vi "Main.vi"(8 "error in (no error)":errorcluster, 11 "LineCCD in":refnum<class "LineCCD.lvclass">) -> (0 "error out":errorcluster, 3 "component":refnum<class "LineCCD.lvclass">)   [LabVIEW 2012, in "LineCCD.lvclass"]
doc: "Main VI of the component. This should contain the GUI of your component and be called when creating an executable."
uses:
  LineCCD.lvclass
  <vilib>/Distrio/Murmex/Murmex/command_enum.ctl
  <instrlib>/ALPHALAS CCD S Series/Public/Typedefs/Operating Mode.ctl
  LineCCD.lvclass/LineCCD.ctl
  <vilib>/Distrio/Murmex/InitialiseMessage/InitialiseMessage.lvclass
  <vilib>/Distrio/Murmex/Murmex/update_cluster.ctl
  <vilib>/Distrio/Murmex/GenericMessage/GenericMessage.lvclass
  <vilib>/Distrio/Murmex/TerminateMessage/TerminateMessage.lvclass
  <vilib>/Distrio/Murmex/ConfigureMessage/ConfigureMessage.lvclass
  <vilib>/Distrio/Murmex/StartMessage/run mode enum.ctl
  <vilib>/Distrio/Murmex/StopMessage/StopMessage.lvclass
  <vilib>/Distrio/Murmex/StartMessage/StartMessage.lvclass
  <vilib>/Distrio/Murmex/ResetMessage/ResetMessage.lvclass
  <vilib>/Distrio/Murmex/Murmex/Set configure at initialise.vi
  <vilib>/Distrio/Murmex/Murmex/Set log reference.vi
  <vilib>/Distrio/Murmex/Murmex/Set VI reference.vi
  <vilib>/Distrio/Murmex/Murmex/Get ID.vi
  <vilib>/Distrio/Murmex/Murmex/Set write log to disk.vi
  <vilib>/Distrio/Murmex/Message/Add or replace parameter.vi
  <vilib>/Distrio/Murmex/Murmex/Murmex.lvclass
  <vilib>/Distrio/Murmex/Message/Message.lvclass
  <instrlib>/ALPHALAS CCD S Series/ALPHALAS CCD S Series.lvlib
panel:
  in  "button:single frame":bool
  in  "Tab Control 2":enum32{"Info"}(tab)
  out "frame rate":dbl[unit]
  out "sensor read out time":dbl[unit]
  out "pixels per scan":u32
  out "pixel height":dbl[unit]
  out "pixel width":dbl[unit]
  out "pixel pitch":dbl[unit]
  out "clock speed":dbl[unit]
  out "trigger out control supported":bool
  out "status":string
  in  "button:reset":bool
  out "terminate?":bool
  in  "Tab Control":enum32{"Main", "Debug"}(tab)
  in  "fit data?":bool
  out "delta":dbl[unit]
  in  "Operating Mode":T1 items=["Int Synch, Continuously Running w SW Capture-Start", "Int Synch, Continuously Running w HW Capture-Start", "Int Synch, Continuously Running w HW Capture-Enable", "Single Shot, Clean&Ready w ext. HW Trigger", "Ext Synch, Continuously Runnung w SW Capture-Start"]
  in  "reset background":bool
  in  "background":bool
  out "max":dbl[unit]
  out "max":u32
  out "min integration time":dbl[unit] caption="min"
  out "max integration time":dbl[unit] caption="max"
  in  "calculate average":bool
  in  "Hardware dark \ncorrection":bool
  in  "Enable trig out\nafter config":bool
  in  "Trig out before integration":dbl[unit] max=0.001849
  in  "Scans per Acquisition":u32 max=4599
  in  "Integration time":dbl[unit] min=9.999999999999999e-06 max=60.0 step=1e-06
  out "Line profile":cluster{cdb[]}[](graph)
  in  "button:select ROIs":bool
  in  "button:free run":bool
  in  "save average":bool
  in  "file name":string
  in  "set intercept":bool
  in  "send delta":bool
  out "pixel shift":dbl
  in  "button:configure":bool
  in  "button:quit":bool
  out "LPB":cluster{cdb[]}[](graph)
  out "LPA":cluster{cdb[]}[](graph)
  out "fitting fine?":bool
  out "signal above threshold?":bool
  in  "Component id":string="LineCCD"
  out "log":string
  in  "button:send command":bool
  in  "generic command":string
  in  "command":T2
  # "Settings"
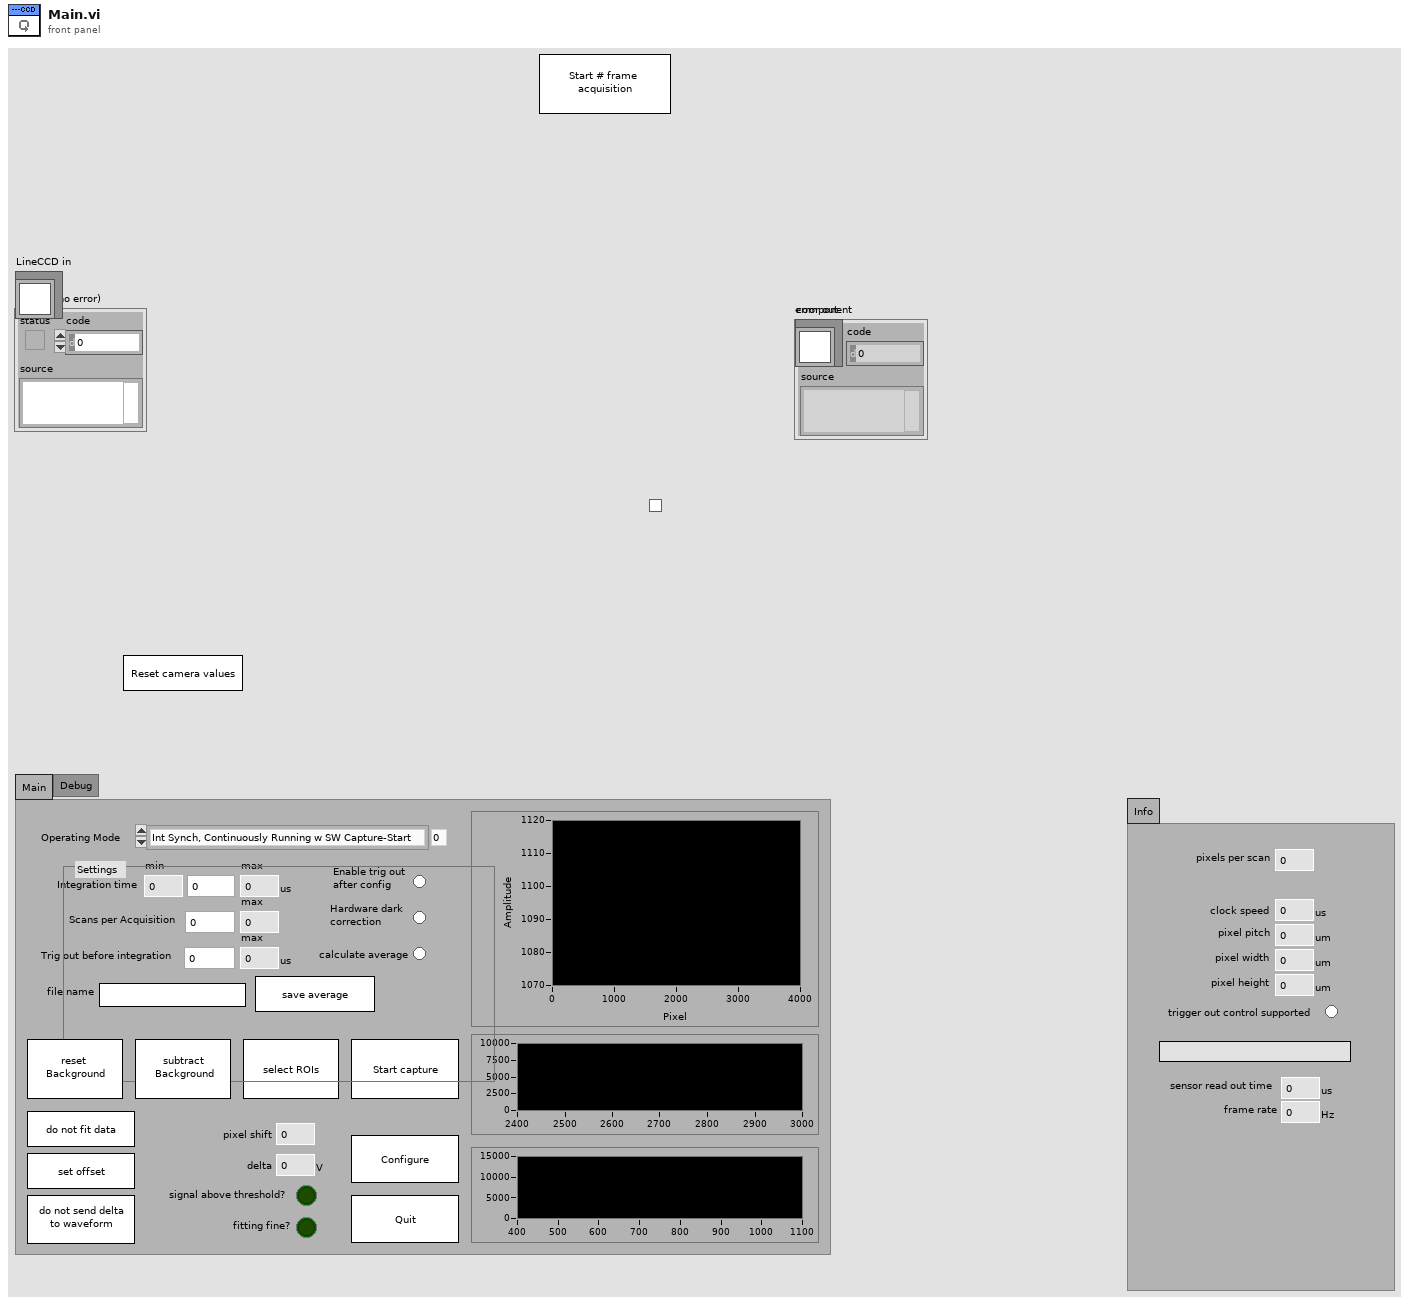
[diagram p1: front panel]
types:
  T1 = typedef "ALPHALAS CCD S Series.lvlib/Operating Mode.ctl" = u16
  T2 = typedef "Murmex.lvlib/Murmex.lvclass/command_enum.ctl" = enum16{"null", "initialise", "reset", "terminate", "acknowledge", "update", "inspect", "inform", "proceed", "start", "stop", "fetch", "configure", "generic"}
  T3 = typedef "Murmex.lvlib/Murmex.lvclass/update_cluster.ctl" = cluster{"target ID":string, "key chains":string[], "values":variant[]}
  T4 = enum8{"Enabled", "Disabled", "Disabled and Grayed Out"}
  T5 = typedef "Murmex.lvlib/StartMessage.lvclass/run mode enum.ctl" = enum16{"infinite", "finite"}
  T6 = typedef "Murmex.lvclass/command_enum.ctl" = enum16{"null", "initialise", "reset", "terminate", "acknowledge", "update", "inspect", "inform", "proceed", "start", "stop", "fetch", "configure", "generic"}
  T7 = typedef "Murmex.lvclass/Event type enumerations.ctl" = enum16{"before", "after"}
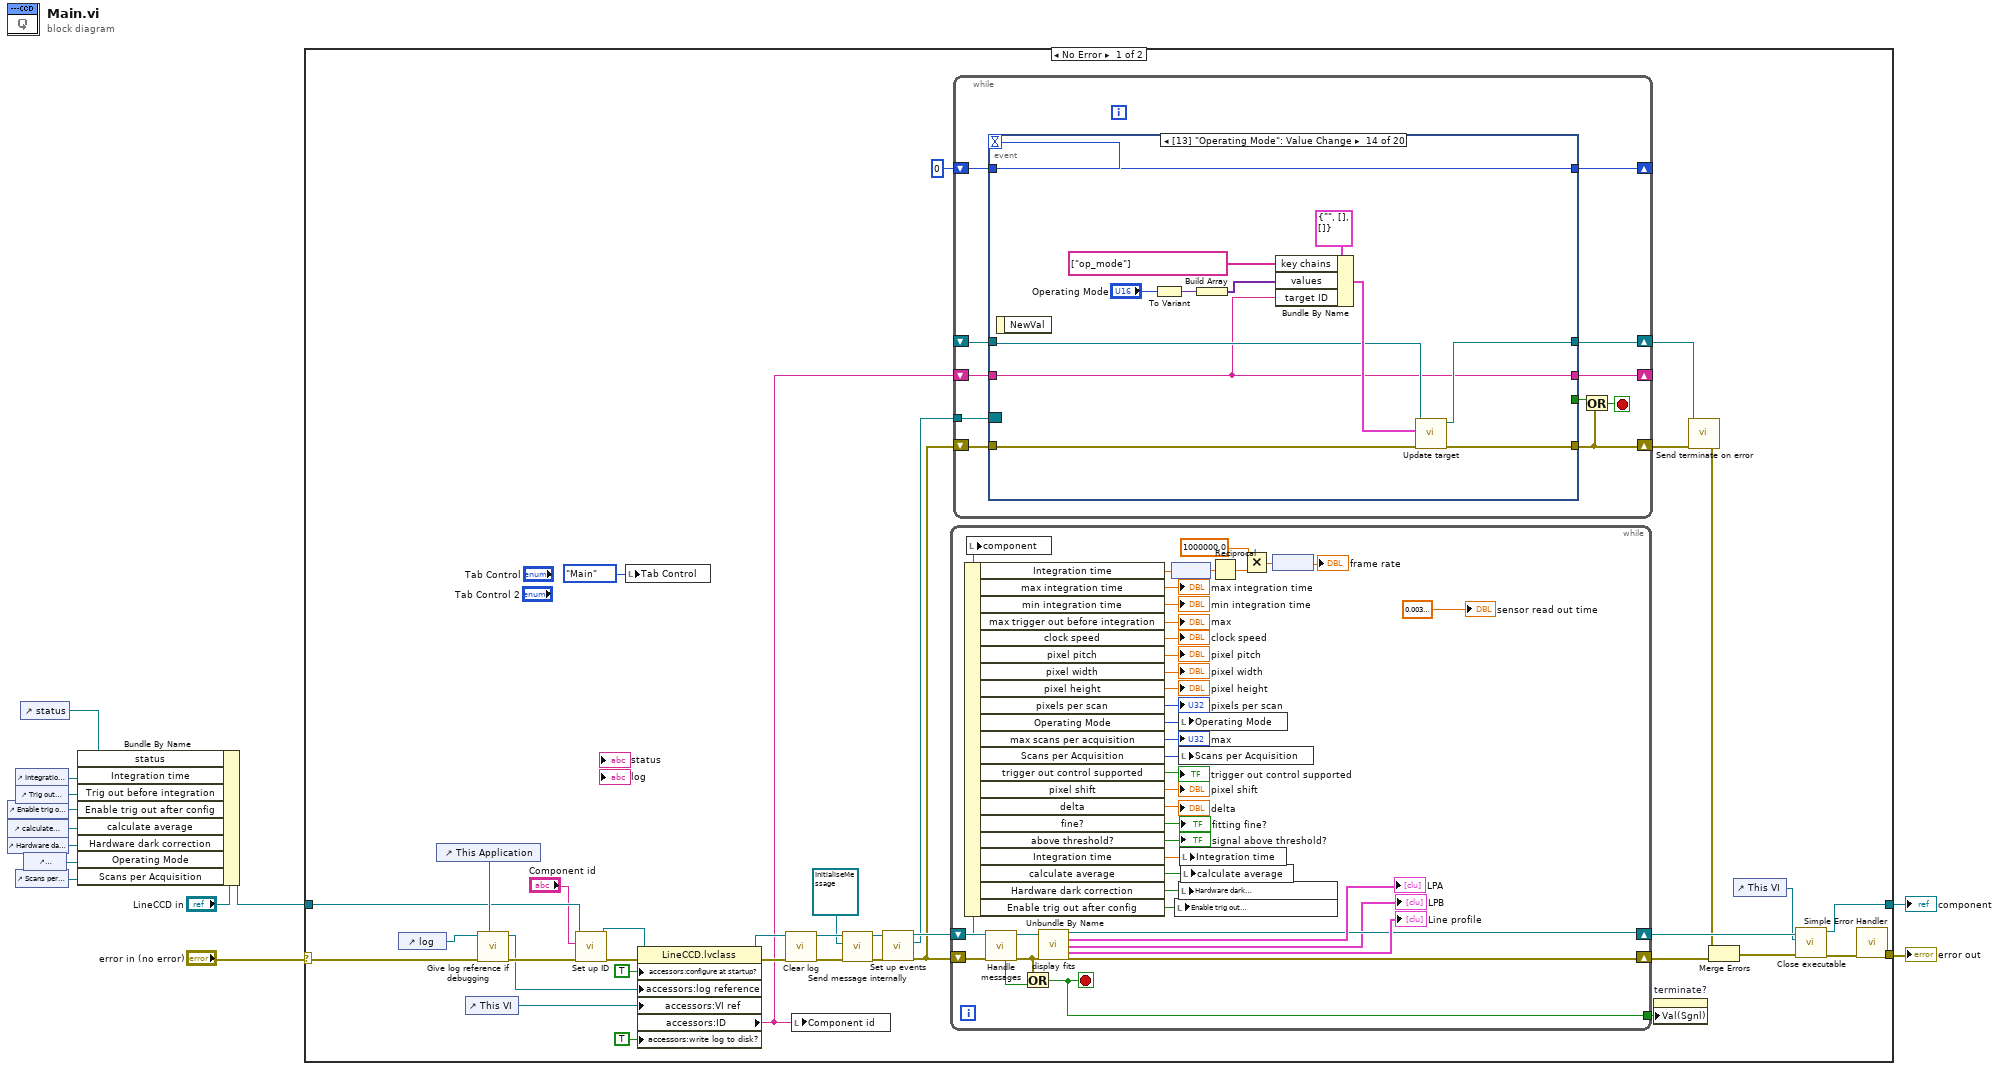
[diagram p0: block diagram]
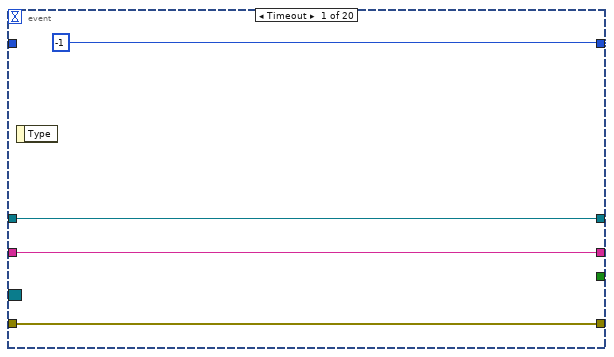
[diagram p2: hidden frame]
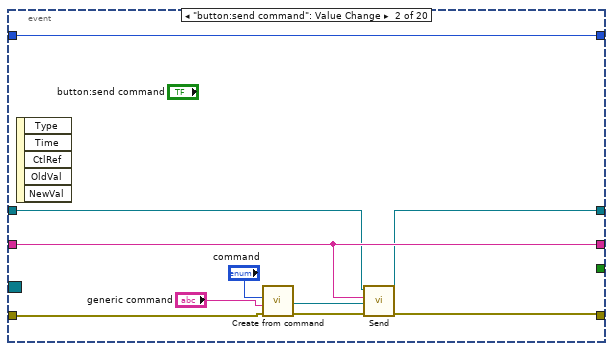
[diagram p3: hidden frame]
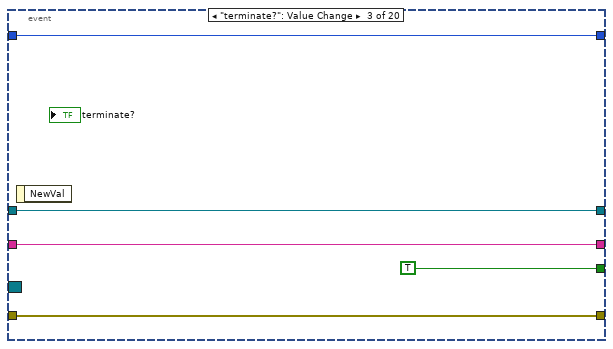
[diagram p4: hidden frame]
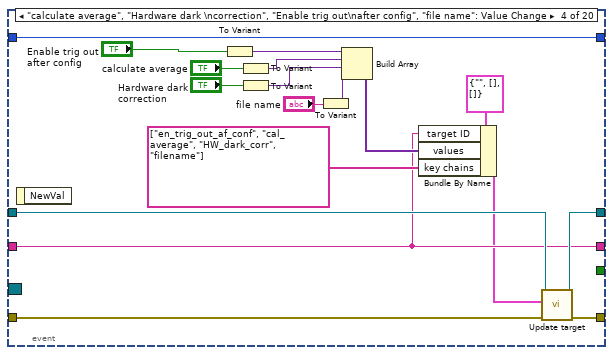
[diagram p5: hidden frame]
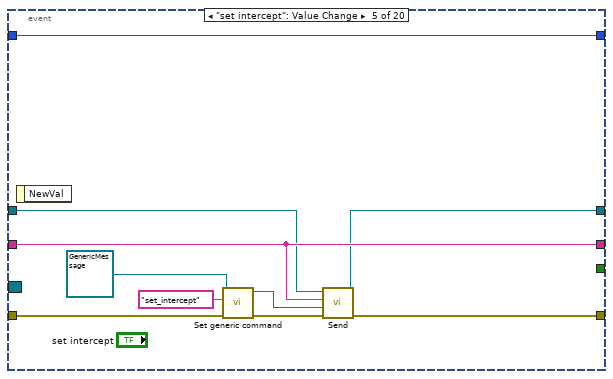
[diagram p6: hidden frame]
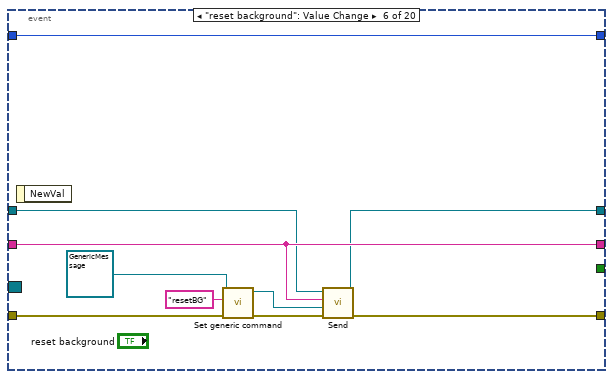
[diagram p7: hidden frame]
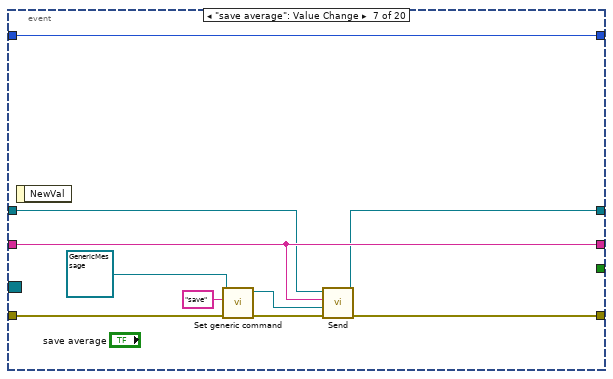
[diagram p8: hidden frame]
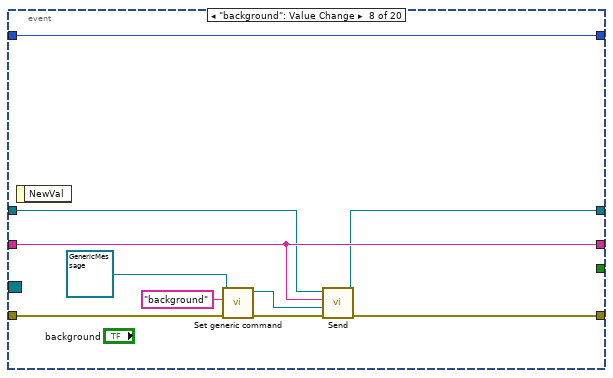
[diagram p9: hidden frame]
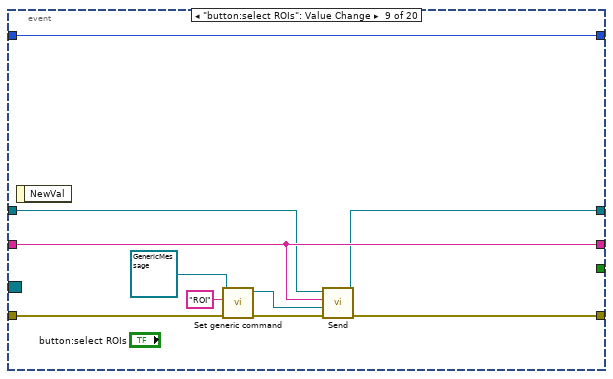
[diagram p10: hidden frame]
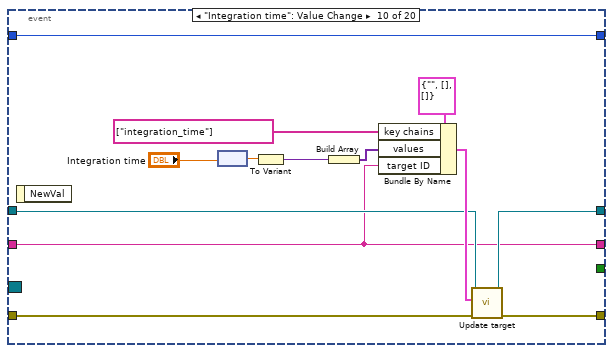
[diagram p11: hidden frame]
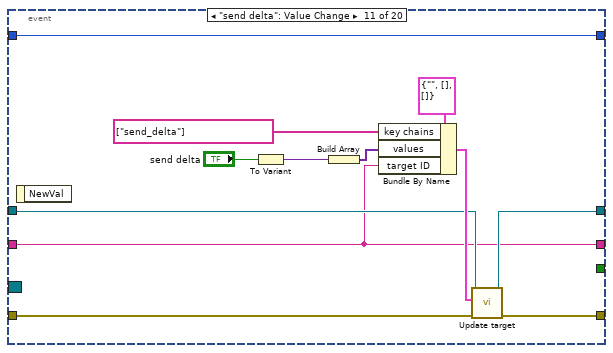
[diagram p12: hidden frame]
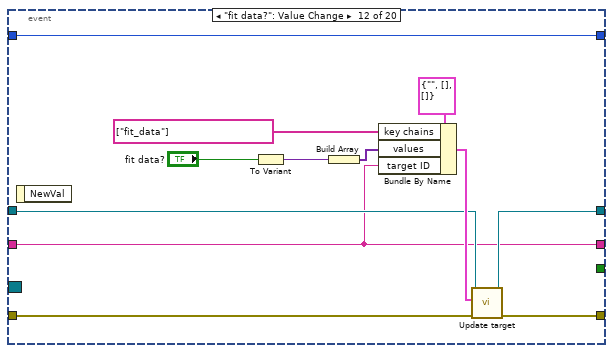
[diagram p13: hidden frame]
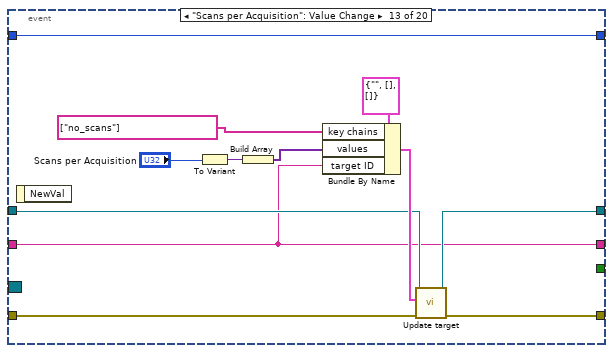
[diagram p14: hidden frame]
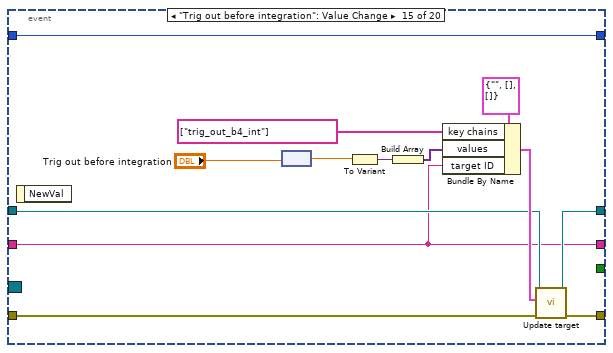
[diagram p15: hidden frame]
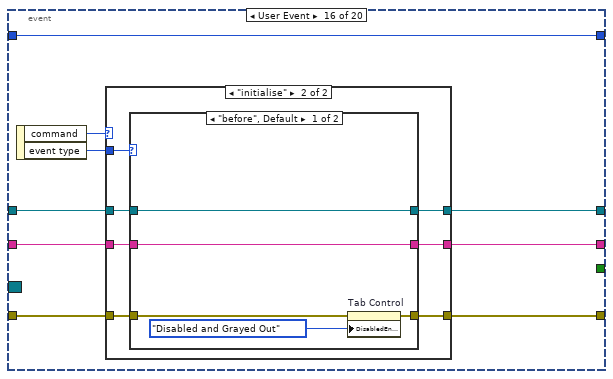
[diagram p16: hidden frame]
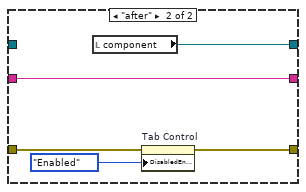
[diagram p18: hidden frame]
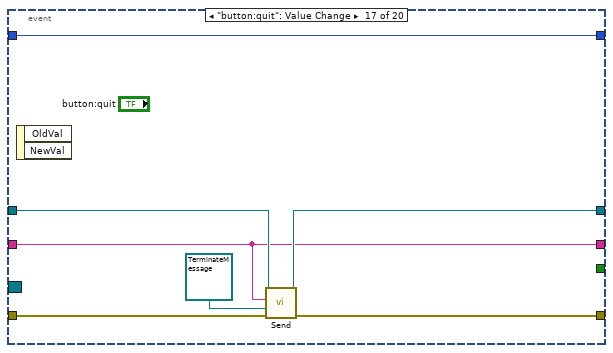
[diagram p19: hidden frame]
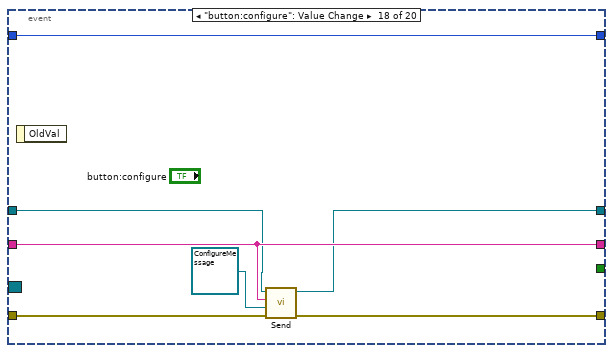
[diagram p20: hidden frame]
diagram:
  n1 = control-ref of="Enable trig out\nafter config"() -> (w5:refnum<vi>)
  n2 = control-ref of="calculate average"() -> (w6:refnum<vi>)
  n3 = control-ref of="Hardware dark \ncorrection"() -> (w7:refnum<vi>)
  n4 = control-ref of="Integration time"() -> (w3:refnum<vi>)
  n5 = control-ref of="Trig out before integration"() -> (w4:refnum<vi>)
  n6 = control-ref of="Scans per Acquisition"() -> (w8:refnum<vi>)
  n7 = control-ref of="status"() -> (w2:refnum<vi>)
  n8 = control-ref of="Operating Mode"() -> (w1:refnum<vi>)
  n9 = Bundle By Name(cluster="LineCCD in", "status"=w2, "Integration time"=w3, "Trig out before integration"=w4, "Enable trig out after config"=w5, "calculate average"=w6, "Hardware dark correction"=w7, "Operating Mode"=w1, "Scans per Acquisition"=w8) -> (w11:refnum<class "LineCCD.lvclass">)
  n10 = case shown="No Error" "error in (no error)" {
    selector: "error in (no error)" -> [w49 w338]
    tunnel: w11 -> [w46 w337]
    tunnel: [w25 w337] -> w10
    tunnel: [w24 w338] -> w9
    frame No Error {
      n11 = control-ref of="log"() -> (w15:refnum<vi>)
      n12 = control-ref of="This Application"() -> (w48:refnum<vi>)
      n13 = control-ref of="This VI"() -> (w41:refnum<vi>)
      n14 = call "Give log reference if debugging.vi"("application ref"=w48, "error in (no error)"=w49, "log reference in"=w15) -> ("error out"=w47:errorcluster, "log reference out"=w42:refnum<vi>)  [unwired: 6 in, 1 out]
      n15 = call <vilib>:"Set up ID.vi"("error in (no error)"=w47, "component ID"="Component id", "MurmexBase in"=w46) -> ("error out"=w45:errorcluster, "MurmexBase out"=w44:refnum<class "LineCCD.lvclass">)  [unwired: 6 in, 1 out]
      n16 = local write "Tab Control"(enum32{"Main", "Debug"}."Main" ("Tab Control")) -> ()
      n17 = property class="LineCCD.lvclass"(reference=w44, error in=w45, "accessors:configure at startup?"=TRUE ("configure at startup?"), "accessors:log reference"=w42, "accessors:VI ref"=w41, "accessors:write log to disk?"=TRUE ("write log to disk?")) -> (reference out=w32:refnum<class "LineCCD.lvclass">, error out=w33:errorcluster, "accessors:ID"=w23:string)
      n18 = call <vilib>:"Clear log.vi"("error in (no error)"=w33, "MurmexBase in"=w32) -> ("error out"=w37:errorcluster, "MurmexBase out"=w38:refnum<class "LineCCD.lvclass">)  [unwired: 8 in]
      n19 = local write "Component id"(w23) -> ()
      n20 = call <vilib>:"Send message internally.vi"("error in (no error)"=w37, "Message"=refnum<class "InitialiseMessage.lvclass"> refnum ("InitialiseMessage"), "Murmex in"=w38) -> ("error out"=w35:errorcluster, "Murmex out"=w34:refnum<class "LineCCD.lvclass">)  [unwired: 7 in]
      n21 = call <vilib>:"Set up events.vi"("error in (no error)"=w35, "MurmexBase in"=w34) -> ("error out"=w22:errorcluster, "Event Registration Refnum"=w21:refnum<event-registration>, "MurmexBase out"=w31:refnum<class "LineCCD.lvclass">)  [unwired: 7 in]
      n22 = while {
        shift-right: [w318] -> w28
        shift-left: w22 -> [w336]
        shift-right: [w319] -> w27
        shift-left: w31 -> [w335]
        tunnel: [w333] -> w17
        stop <- w333 stop-if-true
        n23 = call <vilib>:"Handle messages.vi"("error in (no error)"=w336, "Murmex in"=w335) -> ("error out"=w323:errorcluster, "Murmex out"=w322:refnum<class "LineCCD.lvclass">, "terminated?"=w334:bool)  [unwired: 7 in]
        n24 = Unbundle By Name(w322) -> ("Integration time"=w315:dbl[unit], "max integration time"=→"max integration time":dbl[unit], "min integration time"=→"min integration time":dbl[unit], "max trigger out before integration"=→"max":dbl[unit], "clock speed"=→"clock speed":dbl[unit], "pixel pitch"=→"pixel pitch":dbl[unit], "pixel width"=→"pixel width":dbl[unit], "pixel height"=→"pixel height":dbl[unit], "pixels per scan"=→"pixels per scan":u32, "Operating Mode"=w303:T1, "max scans per acquisition"=→"max":u32, "Scans per Acquisition"=w304:u32, "trigger out control supported"=→"trigger out control supported":bool, "pixel shift"=→"pixel shift":dbl, "delta"=→"delta":dbl[unit], "fine?"=→"fitting fine?":bool, "above threshold?"=→"signal above threshold?":bool, "Integration time"=w302:dbl[unit], "calculate average"=w300:bool, "Hardware dark correction"=w299:bool, "Enable trig out after config"=w301:bool)
        n25 = local write "component"(w322) -> ()
        n26 = Or(x=w323, y=w334) -> (x .or. y?=w333:bool)
        n27 = call-dynamic "display fits.vi"("LineCCD in"=w322, "error in (no error)"=w323) -> ("LPA"=→"LPA":cluster{cdb[]}[], "LineCCD out"=w319:refnum<class "LineCCD.lvclass">, "LPB"=→"LPB":cluster{cdb[]}[], "Line profile"=→"Line profile":cluster{cdb[]}[], "error out"=w318:errorcluster)  [unwired: 13 in]
        n28 = node(w315) -> (w313:dbl)
        n29 = local write "Enable trig out\nafter config"(w301) -> ()
        n30 = local write "Operating Mode"(w303) -> ()
        n31 = local write "Scans per Acquisition"(w304) -> ()
        n32 = local write "Hardware dark \ncorrection"(w299) -> ()
        n33 = local write "Integration time"(w302) -> ()
        n34 = local write "calculate average"(w300) -> ()
        n35 = Reciprocal(x=w313) -> (1/x=w314:dbl)
        n36 = Multiply(x=1000000.0, y=w314) -> (x*y=w312:dbl)
        n37 = node(w312) -> (→"frame rate":dbl[unit])
        "sensor read out time" <- dbl[unit] 0.0037099999999999998 ("sensor read out time")
      }
      n38 = while {
        shift-right: [w54] -> w19
        shift-left: w22 -> [w58]
        tunnel: w21 -> [w52]
        shift-right: [w56] -> _
        shift-left: w23 -> [w57]
        shift-right: [w59] -> _
        shift-left: 0 -> [w60]
        shift-right: [w51] -> w16
        shift-left: _ -> [w50]
        stop <- w53 stop-if-true
        n39 = event shown="[13] \"Operating Mode\": Value Change" {
          selector: w52 -> [_ _ _ _ _ _ _ _ _ _ _ _ _ _ _ _ _ _ _ _]
          dyn-events: _ -> [_ _ _ _ _ _ _ _ _ _ _ _ _ _ _ _ _ _ _ _]
          timeout: w60 -> [_ _ _ _ _ _ _ _ _ _ _ _ _ _ _ _ _ _ _ _]
          tunnel: w60 -> [_ w65 w79 w95 w107 w117 w127 w137 w147 w160 w172 w184 w196 w208 w221 w230 w252 w264 w276 w298]
          tunnel: [-1 w65 w79 w95 w107 w117 w127 w137 w147 w160 w172 w184 w196 w208 w221 w230 w252 w264 w276 w298] -> w59
          tunnel: w58 -> [w61 w70 w78 w94 w102 w112 w122 w132 w142 w154 w167 w179 w191 w203 w215 w229 w256 w263 w275 w296]
          tunnel: [w61 w69 w78 w96 w101 w111 w121 w131 w141 w153 w166 w178 w190 w202 w214 w222 w255 w258 w274 w295] -> w54
          tunnel: w57 -> [w62 w68 w77 w83 w100 w110 w120 w130 w140 w150 w163 w175 w187 w199 w211 w228 w251 w261 w271 w294]
          tunnel: [w62 w68 w77 w83 w100 w110 w120 w130 w140 w150 w163 w175 w187 w199 w211 w223 w251 w261 w270 w294] -> w56
          tunnel: [_ _ TRUE _ _ _ _ _ _ _ _ _ _ _ _ _ _ _ _ _] -> w55
          tunnel: [w63 w66 w75 w93 w98 w108 w118 w128 w138 w151 w164 w176 w188 w200 w212 w227 w253 w259 w272 w292] -> w51
          tunnel: w50 -> [w63 w67 w75 w92 w99 w109 w119 w129 w139 w152 w165 w177 w189 w201 w213 w226 w254 w260 w273 w293]
          event Timeout {
            n40 = event-data() -> ()  [unwired: 1 in, 1 out]
          }
          event "button:send command": Value Change {
            n41 = event-data() -> ()  [unwired: 1 in, 5 out]
            n42 = call <vilib>:"Create from command.vi"("error in (no error)"=w70, "generic command"="generic command", "command"="command") -> ("error out"=w71:errorcluster, "Message out"=w74:refnum<class "Message.lvclass">)  [unwired: 7 in]
            n43 = call <vilib>:"Send.vi"("error in (no error)"=w71, "Message"=w74, "recipient"=w68, "Murmex in"=w67) -> ("error out"=w69:errorcluster, "Murmex out"=w66:refnum<class "LineCCD.lvclass">)  [unwired: 6 in]
          }
          event "terminate?": Value Change {
            n44 = event-data() -> ()  [unwired: 1 in, 1 out]
          }
          event "calculate average", "Hardware dark \ncorrection", "Enable trig out\nafter config", "file name": Value Change {
            n45 = event-data() -> ()  [unwired: 1 in, 1 out]
            n46 = To Variant(anything="Enable trig out\nafter config") -> (Variant=w86:variant)
            n47 = To Variant(anything="calculate average") -> (Variant=w85:variant)
            n48 = To Variant(anything="Hardware dark \ncorrection") -> (Variant=w84:variant)
            n49 = To Variant(anything="file name") -> (Variant=w80:variant)
            n50 = Build Array(w86, w85, w84, w80) -> (w90:variant[])
            n51 = Bundle By Name(cluster=T3 {"target ID"="", "key chains"=[], "values"=[]} ("update cluster"), "target ID"=w83, "values"=w90, "key chains"=string[] ["en_trig_out_af_conf", "cal_average", "HW_dark_corr", "filename"]) -> (w82:T3)
            n52 = call <vilib>:"Update target.vi"("error in (no error)"=w94, "update cluster"=w82, "MurmexBase in"=w92) -> ("error out"=w96:errorcluster, "MurmexBase out"=w93:refnum<class "LineCCD.lvclass">)  [unwired: 7 in]
          }
          event "set intercept": Value Change {
            n53 = event-data() -> ()  [unwired: 1 in, 1 out]
            n54 = call <vilib>:"Set generic command.vi"("error in (no error)"=w102, "generic command"="set_intercept", "GenericMessage in"=refnum<class "GenericMessage.lvclass"> refnum ("Distrio Murmex 1.1:GenericMessage")) -> ("error out"=w105:errorcluster, "GenericMessage out"=w106:refnum<class "GenericMessage.lvclass">)  [unwired: 7 in]
            n55 = call <vilib>:"Send.vi"("error in (no error)"=w105, "Message"=w106, "recipient"=w100, "Murmex in"=w99) -> ("error out"=w101:errorcluster, "Murmex out"=w98:refnum<class "LineCCD.lvclass">)  [unwired: 6 in]
          }
          event "reset background": Value Change {
            n56 = event-data() -> ()  [unwired: 1 in, 1 out]
            n57 = call <vilib>:"Set generic command.vi"("error in (no error)"=w112, "generic command"="resetBG", "GenericMessage in"=refnum<class "GenericMessage.lvclass"> refnum ("Distrio Murmex 1.1:GenericMessage")) -> ("error out"=w115:errorcluster, "GenericMessage out"=w116:refnum<class "GenericMessage.lvclass">)  [unwired: 7 in]
            n58 = call <vilib>:"Send.vi"("error in (no error)"=w115, "Message"=w116, "recipient"=w110, "Murmex in"=w109) -> ("error out"=w111:errorcluster, "Murmex out"=w108:refnum<class "LineCCD.lvclass">)  [unwired: 6 in]
          }
          event "save average": Value Change {
            n59 = event-data() -> ()  [unwired: 1 in, 1 out]
            n60 = call <vilib>:"Set generic command.vi"("error in (no error)"=w122, "generic command"="save", "GenericMessage in"=refnum<class "GenericMessage.lvclass"> refnum ("Distrio Murmex 1.1:GenericMessage")) -> ("error out"=w125:errorcluster, "GenericMessage out"=w126:refnum<class "GenericMessage.lvclass">)  [unwired: 7 in]
            n61 = call <vilib>:"Send.vi"("error in (no error)"=w125, "Message"=w126, "recipient"=w120, "Murmex in"=w119) -> ("error out"=w121:errorcluster, "Murmex out"=w118:refnum<class "LineCCD.lvclass">)  [unwired: 6 in]
          }
          event "background": Value Change {
            n62 = event-data() -> ()  [unwired: 1 in, 1 out]
            n63 = call <vilib>:"Set generic command.vi"("error in (no error)"=w132, "generic command"="background", "GenericMessage in"=refnum<class "GenericMessage.lvclass"> refnum ("Distrio Murmex 1.1:GenericMessage")) -> ("error out"=w135:errorcluster, "GenericMessage out"=w136:refnum<class "GenericMessage.lvclass">)  [unwired: 7 in]
            n64 = call <vilib>:"Send.vi"("error in (no error)"=w135, "Message"=w136, "recipient"=w130, "Murmex in"=w129) -> ("error out"=w131:errorcluster, "Murmex out"=w128:refnum<class "LineCCD.lvclass">)  [unwired: 6 in]
          }
          event "button:select ROIs": Value Change {
            n65 = event-data() -> ()  [unwired: 1 in, 1 out]
            n66 = call <vilib>:"Set generic command.vi"("error in (no error)"=w142, "generic command"="ROI", "GenericMessage in"=refnum<class "GenericMessage.lvclass"> refnum ("Distrio Murmex 1.1:GenericMessage")) -> ("error out"=w145:errorcluster, "GenericMessage out"=w146:refnum<class "GenericMessage.lvclass">)  [unwired: 7 in]
            n67 = call <vilib>:"Send.vi"("error in (no error)"=w145, "Message"=w146, "recipient"=w140, "Murmex in"=w139) -> ("error out"=w141:errorcluster, "Murmex out"=w138:refnum<class "LineCCD.lvclass">)  [unwired: 6 in]
          }
          event "Integration time": Value Change {
            n68 = event-data() -> ()  [unwired: 1 in, 1 out]
            n69 = node("Integration time") -> (w159:dbl)
            n70 = To Variant(anything=w159) -> (Variant=w157:variant)
            n71 = Build Array(w157) -> (w158:variant[])
            n72 = Bundle By Name(cluster=T3 {"target ID"="", "key chains"=[], "values"=[]} ("update cluster"), "key chains"=string[] ["integration_time"], "values"=w158, "target ID"=w150) -> (w156:T3)
            n73 = call <vilib>:"Update target.vi"("error in (no error)"=w154, "update cluster"=w156, "MurmexBase in"=w152) -> ("error out"=w153:errorcluster, "MurmexBase out"=w151:refnum<class "LineCCD.lvclass">)  [unwired: 7 in]
          }
          event "send delta": Value Change {
            n74 = event-data() -> ()  [unwired: 1 in, 1 out]
            n75 = To Variant(anything="send delta") -> (Variant=w170:variant)
            n76 = Build Array(w170) -> (w171:variant[])
            n77 = Bundle By Name(cluster=T3 {"target ID"="", "key chains"=[], "values"=[]} ("update cluster"), "key chains"=string[] ["send_delta"], "values"=w171, "target ID"=w163) -> (w169:T3)
            n78 = call <vilib>:"Update target.vi"("error in (no error)"=w167, "update cluster"=w169, "MurmexBase in"=w165) -> ("error out"=w166:errorcluster, "MurmexBase out"=w164:refnum<class "LineCCD.lvclass">)  [unwired: 7 in]
          }
          event "fit data?": Value Change {
            n79 = event-data() -> ()  [unwired: 1 in, 1 out]
            n80 = To Variant(anything="fit data?") -> (Variant=w182:variant)
            n81 = Build Array(w182) -> (w183:variant[])
            n82 = Bundle By Name(cluster=T3 {"target ID"="", "key chains"=[], "values"=[]} ("update cluster"), "key chains"=string[] ["fit_data"], "values"=w183, "target ID"=w175) -> (w181:T3)
            n83 = call <vilib>:"Update target.vi"("error in (no error)"=w179, "update cluster"=w181, "MurmexBase in"=w177) -> ("error out"=w178:errorcluster, "MurmexBase out"=w176:refnum<class "LineCCD.lvclass">)  [unwired: 7 in]
          }
          event "Scans per Acquisition": Value Change {
            n84 = event-data() -> ()  [unwired: 1 in, 1 out]
            n85 = To Variant(anything="Scans per Acquisition") -> (Variant=w194:variant)
            n86 = Build Array(w194) -> (w195:variant[])
            n87 = Bundle By Name(cluster=T3 {"target ID"="", "key chains"=[], "values"=[]} ("update cluster"), "key chains"=string[] ["no_scans"], "values"=w195, "target ID"=w187) -> (w193:T3)
            n88 = call <vilib>:"Update target.vi"("error in (no error)"=w191, "update cluster"=w193, "MurmexBase in"=w189) -> ("error out"=w190:errorcluster, "MurmexBase out"=w188:refnum<class "LineCCD.lvclass">)  [unwired: 7 in]
          }
          event Value Change {
            n89 = event-data() -> ()  [unwired: 1 in, 1 out]
            n90 = To Variant(anything="Operating Mode") -> (Variant=w206:variant)
            n91 = Build Array(w206) -> (w207:variant[])
            n92 = Bundle By Name(cluster=T3 {"target ID"="", "key chains"=[], "values"=[]} ("update cluster"), "key chains"=string[] ["op_mode"], "values"=w207, "target ID"=w199) -> (w205:T3)
            n93 = call <vilib>:"Update target.vi"("error in (no error)"=w203, "update cluster"=w205, "MurmexBase in"=w201) -> ("error out"=w202:errorcluster, "MurmexBase out"=w200:refnum<class "LineCCD.lvclass">)  [unwired: 7 in]
          }
          event "Trig out before integration": Value Change {
            n94 = event-data() -> ()  [unwired: 1 in, 1 out]
            n95 = node("Trig out before integration") -> (w220:dbl)
            n96 = To Variant(anything=w220) -> (Variant=w218:variant)
            n97 = Build Array(w218) -> (w219:variant[])
            n98 = Bundle By Name(cluster=T3 {"target ID"="", "key chains"=[], "values"=[]} ("update cluster"), "key chains"=string[] ["trig_out_b4_int"], "values"=w219, "target ID"=w211) -> (w217:T3)
            n99 = call <vilib>:"Update target.vi"("error in (no error)"=w215, "update cluster"=w217, "MurmexBase in"=w213) -> ("error out"=w214:errorcluster, "MurmexBase out"=w212:refnum<class "LineCCD.lvclass">)  [unwired: 7 in]
          }
          event User Event {
            n100 = event-data() -> ("command"=w225:T6, "event type"=w224:T7)  [unwired: 1 in]
            n101 = case shown="\"initialise\"" w225 {
              tunnel: w224 -> [_ w240]
              tunnel: w229 -> [w231 w239]
              tunnel: w228 -> [w232 w238]
              tunnel: [w232 w237] -> w223
              tunnel: [w233 w236] -> w227
              tunnel: w226 -> [w233 w235]
              tunnel: [w231 w234] -> w222
              frame "null", Default {
              }
              frame "initialise" {
                n102 = case shown="\"before\", Default" w240 {
                  tunnel: w239 -> [w242 w250]
                  tunnel: [w241 w248] -> w234
                  tunnel: [w244 w247] -> w237
                  tunnel: w238 -> [w244 w247]
                  tunnel: [w245 w246] -> w236
                  tunnel: w235 -> [w245 _]
                  frame "before", Default {
                    n103 = property on="Tab Control" class="TabCtl (strict)"(error in=w242, "DisabledEnum"=T4."Disabled and Grayed Out" ("Disabled")) -> (error out=w241:errorcluster)  [unwired: 1 in, 1 out]
                  }
                  frame "after" {
                    n104 = local read "component"() -> (w246:refnum<class "LineCCD.lvclass">)
                    n105 = property on="Tab Control" class="TabCtl (strict)"(error in=w250, "DisabledEnum"=T4."Enabled" ("Disabled")) -> (error out=w248:errorcluster)  [unwired: 1 in, 1 out]
                  }
                }
              }
            }
          }
          event "button:quit": Value Change {
            n106 = event-data() -> ()  [unwired: 1 in, 2 out]
            n107 = call <vilib>:"Send.vi"("error in (no error)"=w256, "Message"=refnum<class "TerminateMessage.lvclass"> refnum ("TerminateMessage"), "recipient"=w251, "Murmex in"=w254) -> ("error out"=w255:errorcluster, "Murmex out"=w253:refnum<class "LineCCD.lvclass">)  [unwired: 6 in]
          }
          event "button:configure": Value Change {
            n108 = event-data() -> ()  [unwired: 1 in, 1 out]
            n109 = call <vilib>:"Send.vi"("error in (no error)"=w263, "Message"=refnum<class "ConfigureMessage.lvclass"> refnum ("ConfigureMessage"), "recipient"=w261, "Murmex in"=w260) -> ("error out"=w258:errorcluster, "Murmex out"=w259:refnum<class "LineCCD.lvclass">)  [unwired: 6 in]
          }
          event "button:free run": Value Change {
            n110 = event-data() -> ("NewVal"=w265:bool)  [unwired: 1 in]
            n111 = Select(t=run_mode_enum."infinite" ("run mode"), s="button:free run", f=run_mode_enum."finite" ("run mode")) -> (s? t:f=w269:T5)
            n112 = case "start?" shown="False" w265 {
              tunnel: w275 -> [w282 w286]
              tunnel: [w281 w289] -> w274
              tunnel: w273 -> [w280 w291]
              tunnel: [w279 w290] -> w272
              tunnel: w271 -> [w278 w288]
              tunnel: [w278 w288] -> w270
              tunnel: w269 -> [_ w287]
              frame False {
                n113 = call <vilib>:"Send message internally.vi"("error in (no error)"=w282, "Message"=refnum<class "StopMessage.lvclass"> refnum ("Distrio Murmex 1.5:StopMessage"), "Murmex in"=w280) -> ("error out"=w281:errorcluster, "Murmex out"=w279:refnum<class "LineCCD.lvclass">)  [unwired: 7 in]
              }
              frame True {
                n114 = call <vilib>:"Set run mode.vi"("error in (no error)"=w286, "run mode"=w287, "StartMessage in"=refnum<class "StartMessage.lvclass"> refnum ("Message in")) -> ("error out"=w285:errorcluster, "StartMessage out"=w283:refnum<class "StartMessage.lvclass">)  [unwired: 7 in]
                n115 = call <vilib>:"Send message internally.vi"("error in (no error)"=w285, "Message"=w283, "Murmex in"=w291) -> ("error out"=w289:errorcluster, "Murmex out"=w290:refnum<class "LineCCD.lvclass">)  [unwired: 7 in]
              }
            }
          }
          event "button:reset": Value Change {
            n116 = event-data() -> ()  [unwired: 1 in, 1 out]
            n117 = call <vilib>:"Send message internally.vi"("error in (no error)"=w296, "Message"=refnum<class "ResetMessage.lvclass"> refnum ("Message in"), "Murmex in"=w293) -> ("error out"=w295:errorcluster, "Murmex out"=w292:refnum<class "LineCCD.lvclass">)  [unwired: 7 in]
          }
        }
        n118 = Or(x=w55, y=w54) -> (x .or. y?=w53:bool)
      }
      n119 = property on="terminate?" class="Bool (strict)"("Val(Sgnl)"=w17) -> ()  [unwired: 2 in, 2 out]
      n120 = call <vilib>:"Send terminate on error.vi"("error in (no error)"=w19, "Murmex in"=w16) -> ("error out"=w18:errorcluster)  [unwired: 8 in, 1 out]
      n121 = Merge Errors(w18, w28) -> (w29:errorcluster)
      n122 = control-ref of="This VI"() -> (w26:refnum<vi>)
      n123 = call <vilib>:"Close executable.vi"("error in (no error)"=w29, "main VI ref (optional)"=w26, "MurmexBase in"=w27) -> ("error out"=w30:errorcluster, "MurmexBase out"=w25:refnum<class "LineCCD.lvclass">)  [unwired: 7 in]
      n124 = call <vilib>:"Simple Error Handler.vi"("error in (no error)"=w30) -> ("error out"=w24:errorcluster)  [unwired: 4 in, 4 out]
    }
    frame Error {
    }
  }
  "error out" <- w9
  "component" <- w10
